vi "Configure Display.vi"(6 "Enable Display (on)":bool, 8 "error in (no error)":errorcluster, 9 "display type (meas:0)":u16(ring) items=["measurement display", "comparison display", "limit table display (primary)", "limit table display (secondary)"], 11 "VISA resource name":refnum<visa-resource-name>) -> (0 "error out":errorcluster, 3 "VISA resource name out":refnum<visa-resource-name>)   [LabVIEW 2016, in "Agilent 4263X.lvlib"]
doc: "This VI configures the display mode (for the instrument's display screen only)."
uses:
  <instrlib>/Agilent 4263X/Agilent 4263X.lvlib
panel:
  # "on\noff"
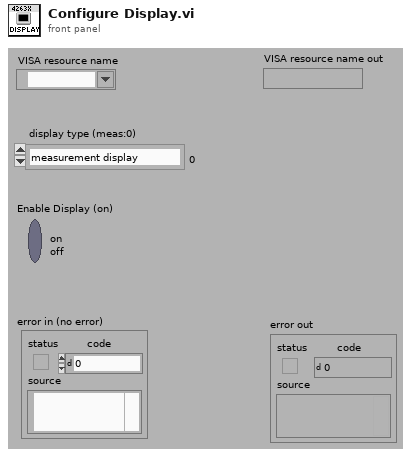
[diagram p1: front panel]
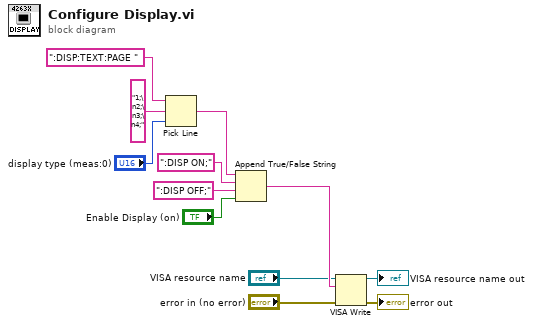
[diagram p0: block diagram]
diagram:
  n1 = Pick Line(string ("")=":DISP:TEXT:PAGE ", multi-line string="1;\n2;\n3;\n4;", line index="display type (meas:0)") -> (output string=w2:string)
  n2 = Append True/False String(1:"Enable Display (on)", 2:":DISP OFF;", 3:":DISP ON;", 4:w2) -> (0:w3:string)
  n3 = VISA Write(VISA resource name="VISA resource name", write buffer=w3, error in (no error)="error in (no error)") -> (VISA resource name out=→"VISA resource name out":refnum<visa-resource-name>, error out=→"error out":errorcluster)  [unwired: 1 out]
